vi "Get_data.vi"() -> (0 "EOF? and Error status":bool, 6 "Block Header":string)   [LabVIEW 2012]
uses:
  Controls/Block_start_and_end.ctl
  Globals/Meas_global.vi
  Globals/LDA_meas_global_1.vi
  Globals/Trav_pos_global.vi
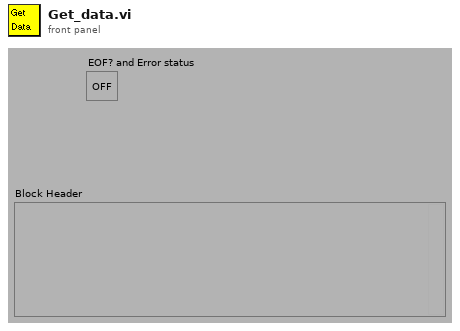
[diagram p1: front panel]
types:
  T1 = typedef "Block_start_and_end.ctl" = cluster{"Started":dbl, "Ended":dbl, "Analogue Frequency Hz":dbl}
  T2 = typedef "Post_Process.ctl" = enum16{"Take New Data", "Post Process Raw Data File"}
  T3 = typedef "PWA_Data.ctl" = enum16{"No PWA Data", "One Ch PWA"}
  T4 = typedef "BSA_Type.ctl" = enum16{"57N11", "BSA F60"}
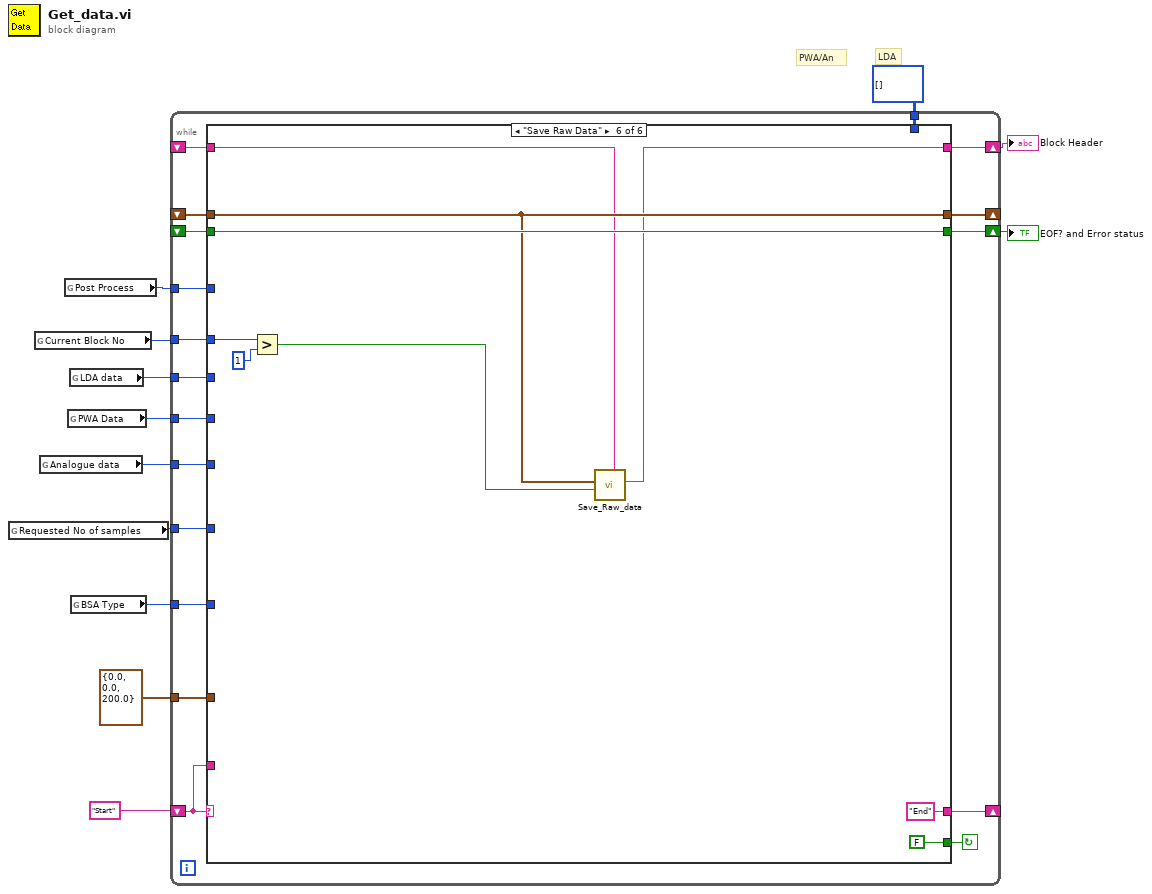
[diagram p0: block diagram]
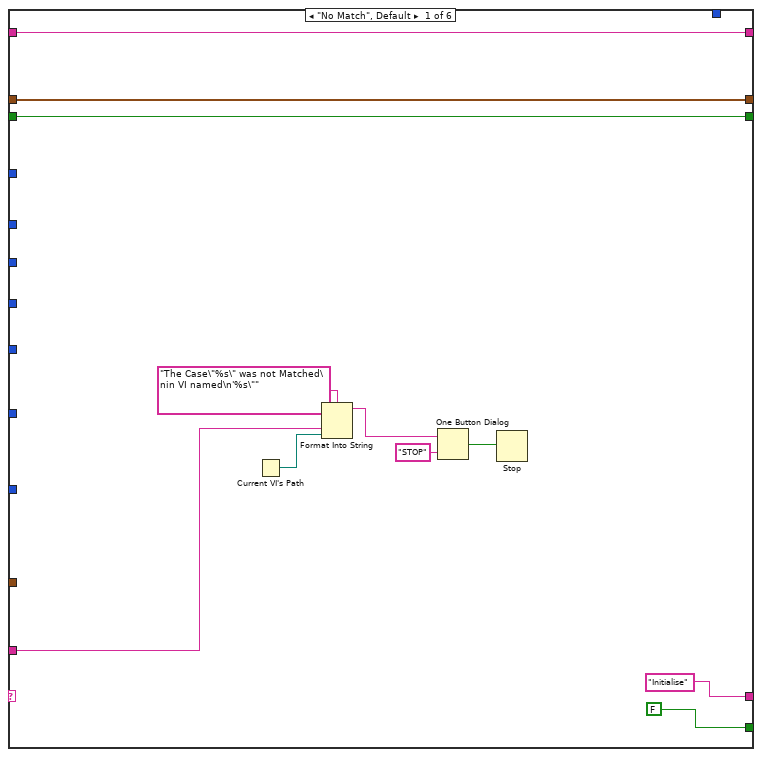
[diagram p2: hidden frame]
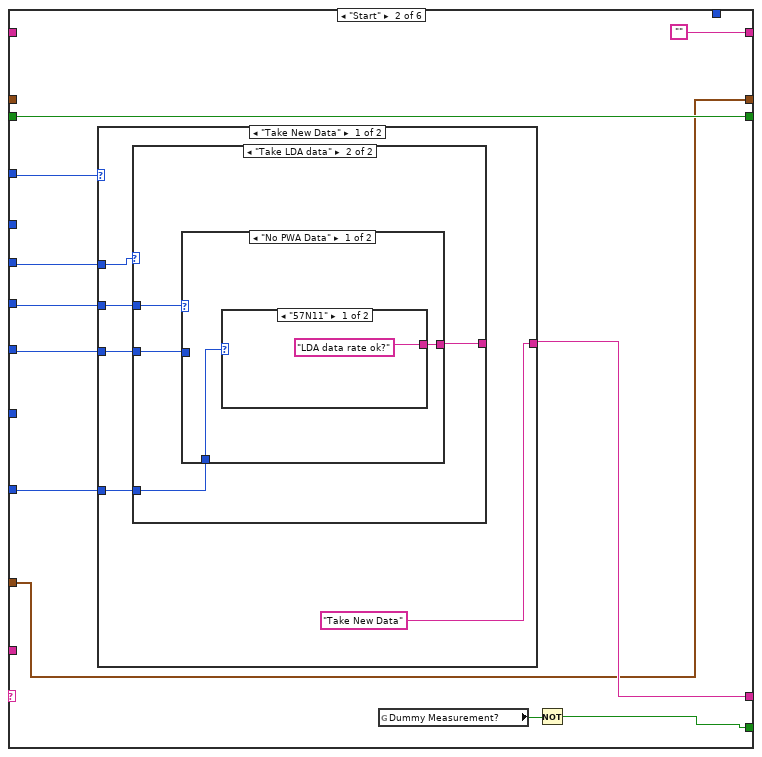
[diagram p3: hidden frame]
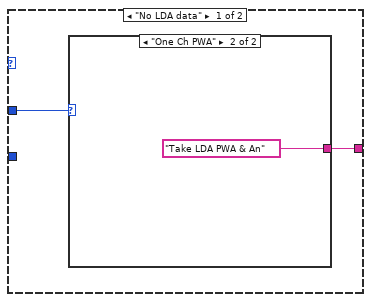
[diagram p4: hidden frame]
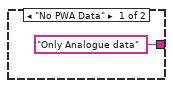
[diagram p5: hidden frame]
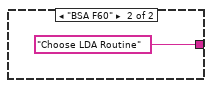
[diagram p6: hidden frame]
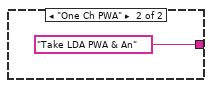
[diagram p7: hidden frame]
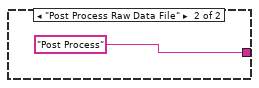
[diagram p8: hidden frame]
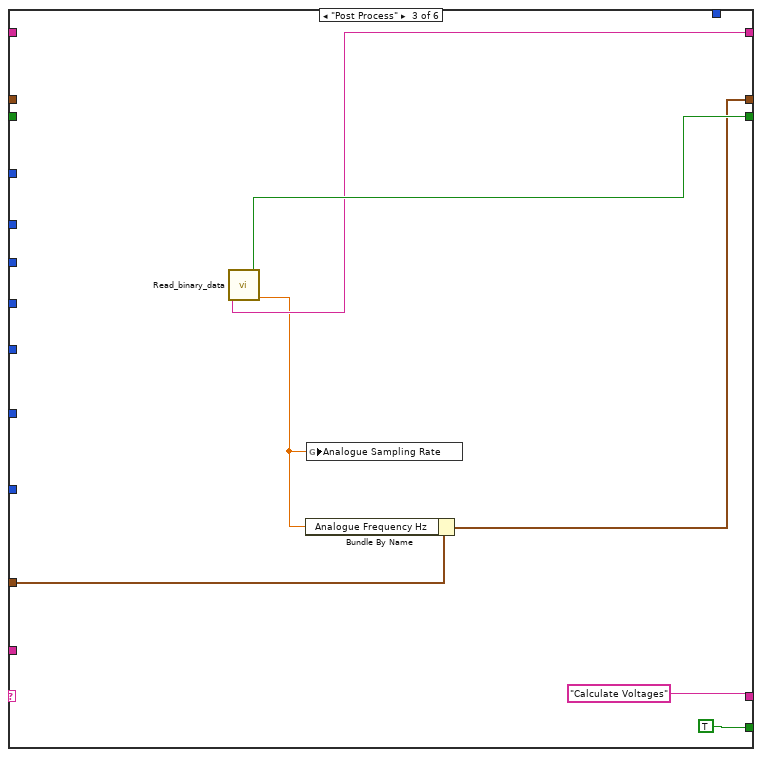
[diagram p9: hidden frame]
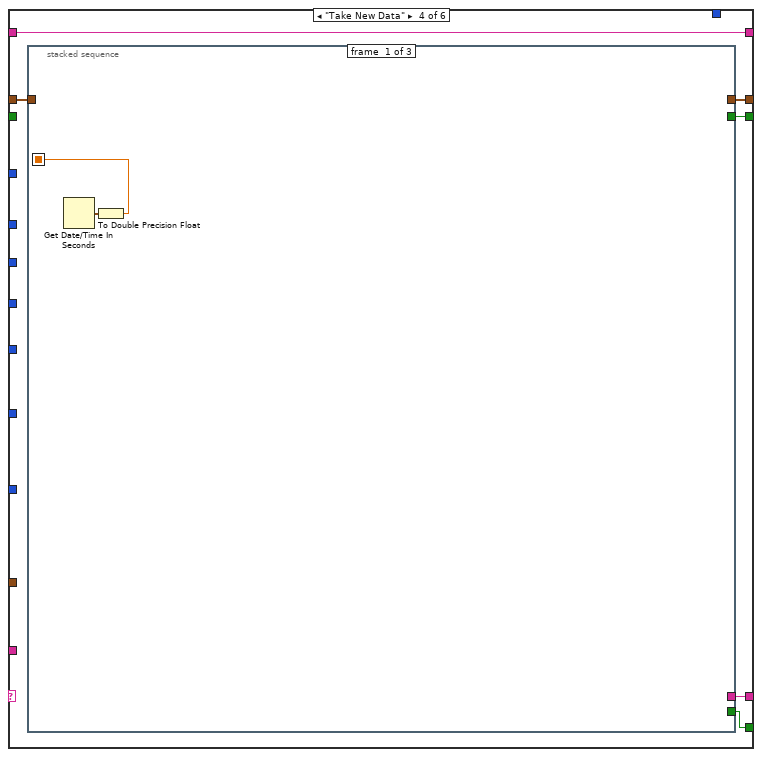
[diagram p10: hidden frame]
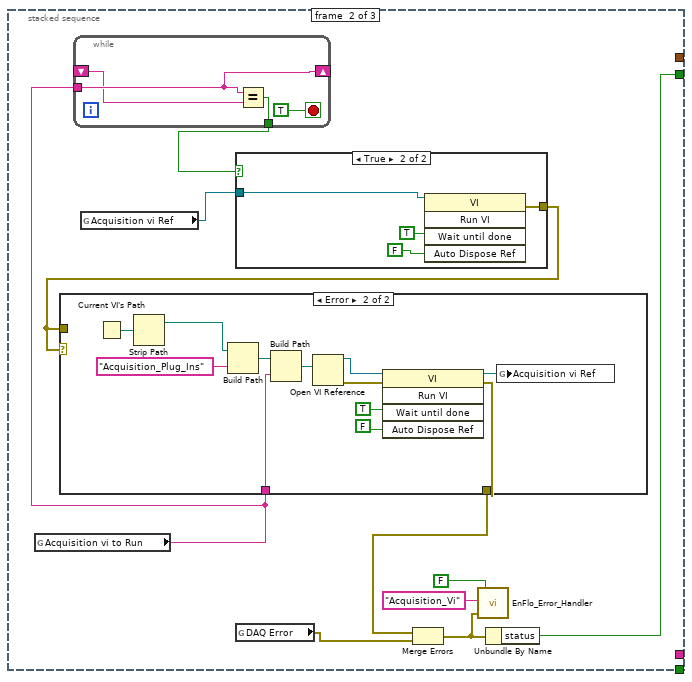
[diagram p11: hidden frame]
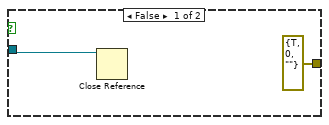
[diagram p12: hidden frame]
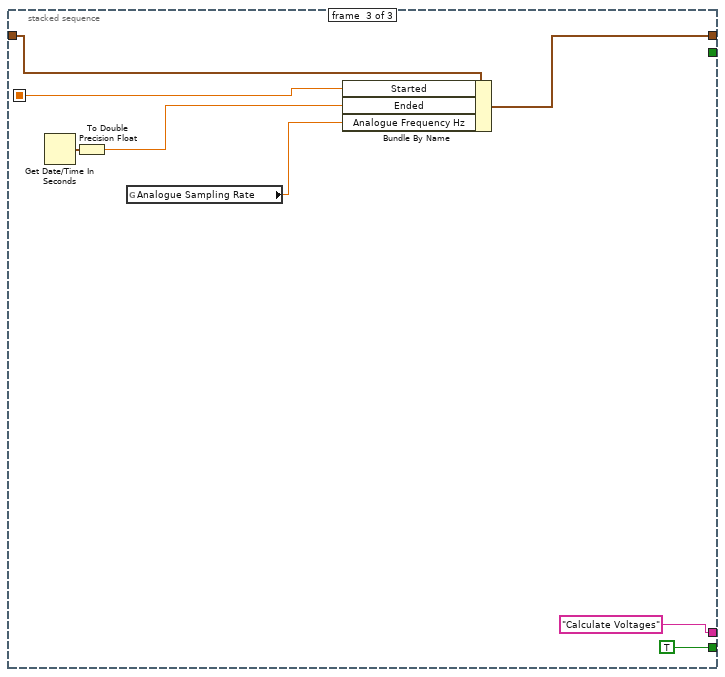
[diagram p14: hidden frame]
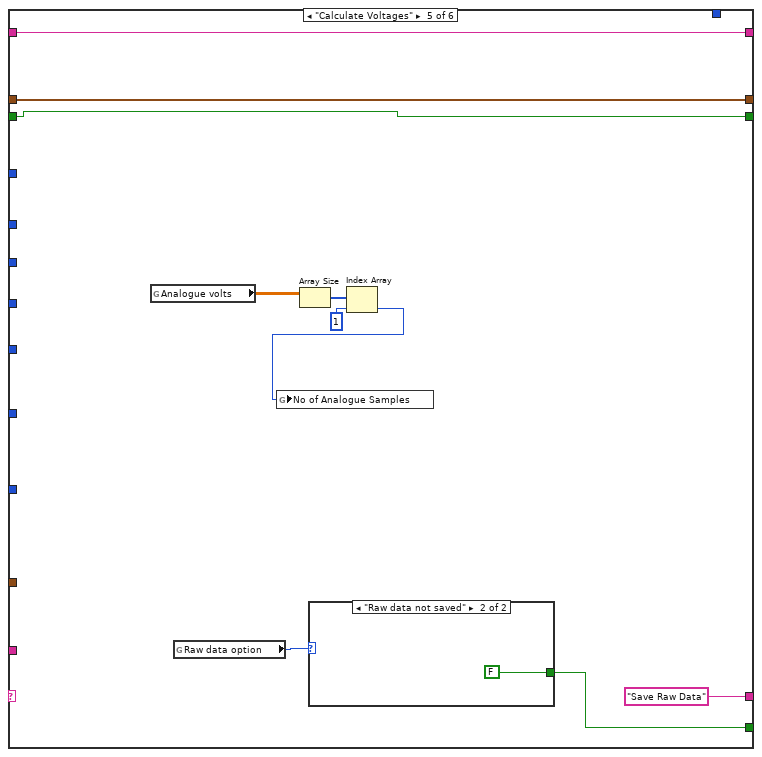
[diagram p15: hidden frame]
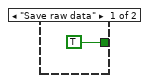
[diagram p16: hidden frame]
diagram:
  # "LDA"
  # "PWA/An"
  n1 = global read "Meas_global.vi" "Requested No of samples"() -> (w8:i32)
  n2 = global read "Meas_global.vi" "Current Block No"() -> (w7:i32)
  n3 = global read "Meas_global.vi" "Analogue data"() -> (w6:enum16{"No Analogue data", "Take Analogue data"})
  n4 = global read "Meas_global.vi" "Post Process"() -> (w9:T2)
  n5 = global read "Meas_global.vi" "PWA Data"() -> (w4:T3)
  n6 = global read "Meas_global.vi" "LDA data"() -> (w5:enum16{"No LDA data", "Take LDA data"})
  n7 = global read "LDA_meas_global_1.vi" "BSA Type"() -> (w1:T4)
  n8 = while {
    shift-left: "Start" -> [w28]
    shift-right: [w29] -> _
    shift-right: [w27] -> _
    shift-left: _ -> [w26]
    shift-right: [w25] -> w11
    shift-left: _ -> [w24]
    tunnel: T1 {"Started"=0.0, "Ended"=0.0, "Analogue Frequency Hz"=200.0} ("Block Timings") -> [w23]
    tunnel: w9 -> [w22]
    tunnel: w8 -> [w21]
    tunnel: w7 -> [w20]
    tunnel: w6 -> [w19]
    tunnel: w5 -> [w18]
    tunnel: w4 -> [w17]
    tunnel: u16[][] [] ("LDA Binary output") -> [w16]
    tunnel: w1 -> [w15]
    shift-right: [w13] -> w2
    shift-left: _ -> [w14]
    stop <- w30 continue-if-true
    n9 = case shown="\"Save Raw Data\"" w28 {
      tunnel: [FALSE w42 TRUE w80 w133 FALSE] -> w30
      tunnel: ["Initialise" w50 "Calculate Voltages" w81 "Save Raw Data" "End"] -> w29
      tunnel: w28 -> [w36 _ _ _ _ _]
      tunnel: [w33 w44 w74 w82 w137 w147] -> w27
      tunnel: w26 -> [w33 _ _ w83 w137 w147]
      tunnel: [w31 w52 w75 w79 w136 w148] -> w25
      tunnel: w24 -> [w31 w52 _ _ w136 w148]
      tunnel: w23 -> [_ w44 w76 _ _ _]
      tunnel: w22 -> [_ w51 _ _ _ _]
      tunnel: w21 -> [_ _ _ _ _ _]
      tunnel: w20 -> [_ _ _ _ _ w142]
      tunnel: w19 -> [_ w49 _ _ _ _]
      tunnel: w18 -> [_ w48 _ _ _ _]
      tunnel: w17 -> [_ w47 _ _ _ _]
      tunnel: w16 -> [_ _ _ _ _ _]
      tunnel: w15 -> [_ w46 _ _ _ _]
      tunnel: [w32 "" w73 w84 w132 w144] -> w13
      tunnel: w14 -> [w32 _ _ w84 w132 w143]
      frame "No Match", Default {
        n10 = Current VI's Path() -> (path=w35:path)
        n11 = Format Into String(format string="The Case\"%s\" was not Matched\nin VI named\n'%s\"" ("Format String"), w36, w35) -> (resulting string=w39:string)  [unwired: 2 in, 1 out]
        n12 = One Button Dialog(message=w39, button name ("OK")="STOP") -> (true=w37:bool)
        n13 = Stop(stop? (T)=w37) -> ()
      }
      frame "Start" {
        n14 = case shown="\"Take New Data\"" w51 {
          tunnel: ["Take New Data" "Post Process"] -> w50
          tunnel: w49 -> [w57 _]
          tunnel: w48 -> [w56 _]
          tunnel: w47 -> [w55 _]
          tunnel: w46 -> [w54 _]
          frame "Take New Data" {
            n15 = case shown="\"Take LDA data\"" w56 {
              tunnel: w57 -> [_ w63]
              tunnel: [w58 w65] -> _
              tunnel: w55 -> [w59 w64]
              tunnel: w54 -> [_ w62]
              frame "No LDA data" {
                n16 = case shown="\"One Ch PWA\"" w59 {
                  tunnel: ["Only Analogue data" "Take LDA PWA & An"] -> w58
                  frame "No PWA Data" {
                  }
                  frame "One Ch PWA" {
                  }
                }
              }
              frame "Take LDA data" {
                n17 = case shown="\"No PWA Data\"" w64 {
                  tunnel: [w66 "Take LDA PWA & An"] -> w65
                  tunnel: w63 -> [_ _]
                  tunnel: w62 -> [w67 _]
                  frame "No PWA Data" {
                    n18 = case shown="\"57N11\"" w67 {
                      tunnel: ["LDA data rate ok?" "Choose LDA Routine"] -> w66
                      frame "57N11" {
                      }
                      frame "BSA F60" {
                      }
                    }
                  }
                  frame "One Ch PWA" {
                  }
                }
              }
            }
          }
          frame "Post Process Raw Data File" {
          }
        }
        n19 = global read "Trav_pos_global.vi" "Dummy Measurement?"() -> (w43:bool)
        n20 = Not(x=w43) -> (.not. x?=w42:bool)
      }
      frame "Post Process" {
        n21 = call "Read_binary_data.vi"() -> ("Analogue Frequency Hz"=w72:dbl, "EOF?"=w75:bool, "Block Header"=w73:string)  [unwired: 7 out]
        n22 = Bundle By Name(cluster=w76, "Analogue Frequency Hz"=w72) -> (w74:T1)
        n23 = global write "Meas_global.vi" "Analogue Sampling Rate"(w72) -> ()
      }
      frame "Take New Data" {
        n24 = stacked-sequence {
          seq-local: [w85 _ _] -> [_ _ w125]
          tunnel: w83 -> [_ _ w126]
          tunnel: [_ _ w123] -> w82
          tunnel: [_ _ "Calculate Voltages"] -> w81
          tunnel: [_ _ TRUE] -> w80
          tunnel: [_ w87 _] -> w79
          frame #0 {
            n25 = Get Date/Time In Seconds() -> (seconds since 1Jan1904=w86:timestamp)
            n26 = To Double Precision Float(number=w86) -> (double precision float=w85:dbl)
          }
          frame #1 {
            n27 = global read "Meas_global.vi" "Acquisition vi to Run"() -> (w94:string)
            n28 = while {
              shift-right: [w106] -> _
              shift-left: _ -> [w105]
              tunnel: w94 -> [w106]
              tunnel: [w103] -> w93
              stop <- TRUE stop-if-true
              n29 = Equal?(x=w106, y=w105) -> (x = y?=w103:bool)
            }
            n30 = global read "Meas_global.vi" "Acquisition vi Ref"() -> (w91:refnum<vi>)
            n31 = case shown="True" w93 {
              tunnel: [errorcluster {"status"=TRUE, "code"=0, "source"=""} ("error out") w100] -> w92
              tunnel: w91 -> [w97 w99]
              frame False {
                n32 = Close Reference(reference=w97) -> ()  [unwired: 1 in, 1 out]
              }
              frame True {
                n33 = invoke class="VI" method="Run VI"(reference=w99, "Wait until done"=TRUE ("Wait Until Done"), "Auto Dispose Ref"=FALSE ("Wait until done")) -> (error out=w100:errorcluster)  [unwired: 2 in, 4 out]
              }
            }
            n34 = case shown="Error" w92 {
              tunnel: [w107 w109] -> w90
              tunnel: w94 -> [_ w108]
              tunnel: w92 -> [w107 _]
              frame No Error {
              }
              frame Error {
                n35 = Current VI's Path() -> (path=w119:path)
                n36 = Strip Path(path=w119) -> (stripped path=w117:path)  [unwired: 1 out]
                n37 = Build Path(base path=w117, name or relative path="Acquisition_Plug_Ins") -> (appended path=w116:path)
                n38 = Build Path(base path=w116, name or relative path=w108) -> (appended path=w115:path)
                n39 = Open VI Reference(vi path=w115) -> (vi reference=w112:refnum<vi>, error out=w111:errorcluster)  [unwired: 5 in]
                n40 = invoke class="VI" method="Run VI"(reference=w112, error in=w111, "Wait until done"=TRUE ("Wait Until Done"), "Auto Dispose Ref"=FALSE ("Wait until done")) -> (reference out=w110:refnum<vi>, error out=w109:errorcluster)  [unwired: 1 in, 3 out]
                n41 = global write "Meas_global.vi" "Acquisition vi Ref"(w110) -> ()
              }
            }
            n42 = global read "Meas_global.vi" "DAQ Error"() -> (w89:errorcluster)
            n43 = Merge Errors(w90, w89) -> (w88:errorcluster)
            n44 = call "EnFlo_Error_Handler.vi"("error in (no error)"=w88, "Error Type"="Acquisition_Vi", "Dialog Box (T)"=FALSE) -> ()  [unwired: 3 out]
            n45 = Unbundle By Name(w88) -> ("status"=w87:bool)
          }
          frame #2 {
            n46 = Get Date/Time In Seconds() -> (seconds since 1Jan1904=w127:timestamp)
            n47 = To Double Precision Float(number=w127) -> (double precision float=w124:dbl)
            n48 = global read "Meas_global.vi" "Analogue Sampling Rate"() -> (w120:dbl)
            n49 = Bundle By Name(cluster=w126, "Started"=w125, "Ended"=w124, "Analogue Frequency Hz"=w120) -> (w123:T1)
          }
        }
      }
      frame "Calculate Voltages" {
        n50 = global read "Meas_global.vi" "Analogue volts"() -> (w128:dbl[][])
        n51 = global read "Meas_global.vi" "Raw data option"() -> (w135:enum16{"Save raw data", "Raw data not saved"})
        n52 = Array Size(array=w128) -> (size(s)=w129:i32[])
        n53 = case shown="\"Raw data not saved\"" w135 {
          tunnel: [TRUE FALSE] -> w133
          frame "Save raw data" {
          }
          frame "Raw data not saved" {
          }
        }
        n54 = Index Array(array=w129, index=1) -> (element=w131:i32)
        n55 = global write "Meas_global.vi" "No of Analogue Samples"(w131) -> ()
      }
      frame "Save Raw Data" {
        n56 = Greater?(x=w142, y=1) -> (0:w140:bool)
        n57 = call "Save_Raw_data.vi"("Add to Block Header"=w143, "append to file? (new file:F)"=w140, "Block Timings"=w147) -> ("Block Header"=w144:string)  [unwired: 6 in]
      }
    }
  }
  "EOF? and Error status" <- w11
  "Block Header" <- w2
